vi "GPS Read Sim. Instance.vi"(0 "String In":string, 1 "Buffer In":string, 5 "error in (no error)":errorcluster) -> (13 "Output Valid":bool, 14 "String Out":string, 15 "Buffer Out":string, 16 "Time":dbl, 17 "Longitude":dbl, 18 "Latitude":dbl, 19 "error out":errorcluster)   [LabVIEW 2009]
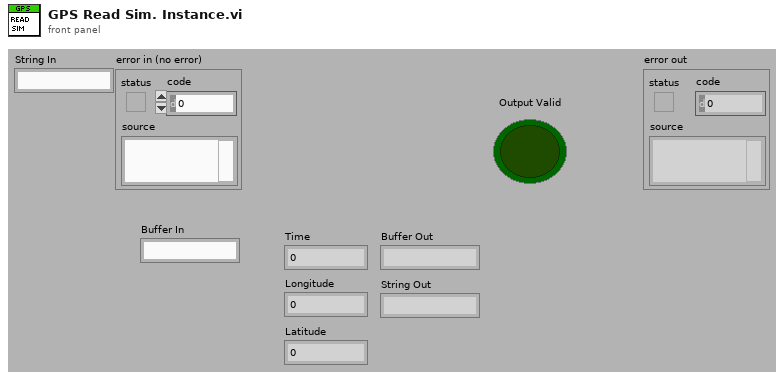
[diagram p1: front panel]
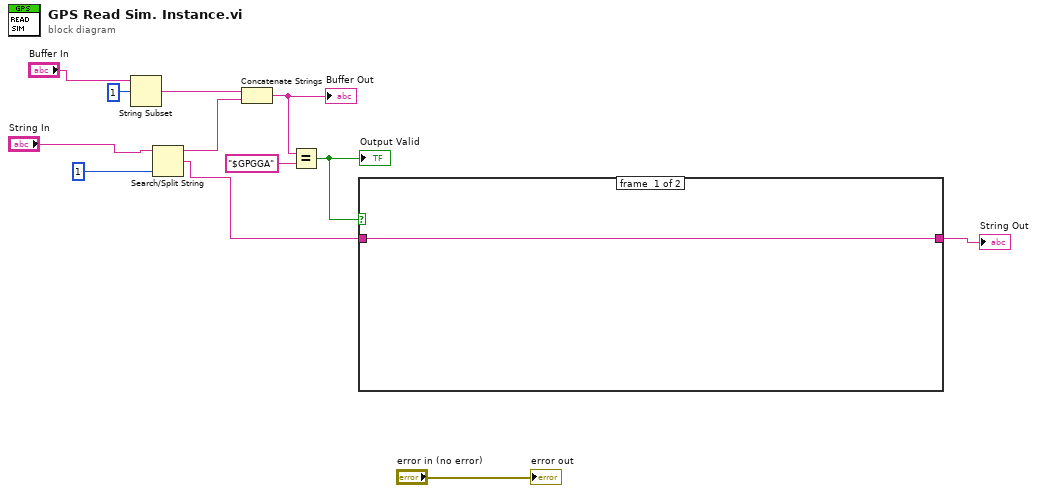
[diagram p0: block diagram]
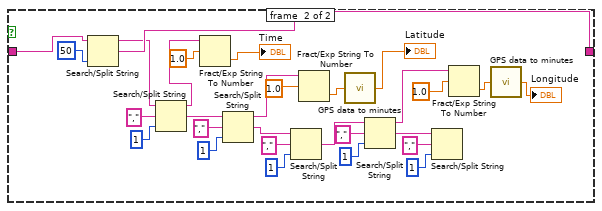
[diagram p2: hidden frame]
diagram:
  n1 = String Subset(string="Buffer In", offset (0)=1) -> (substring=w11:string)  [unwired: 1 in]
  n2 = Search/Split String(string="String In", offset (0)=1 ("length (rest)")) -> (substring before match=w4:string, match + rest of string=w3:string)  [unwired: 1 in, 1 out]
  n3 = Concatenate Strings(w11, w4) -> (w10:string)
  "Buffer Out" <- w10
  n4 = Equal?(x=w10, y="$GPGGA") -> (x = y?=w8:bool)
  "Output Valid" <- w8
  n5 = case shown="True" w8 {
    tunnel: w3 -> [w13 w42]
    tunnel: [w13 w19] -> w2
    frame #0 {
    }
    frame #1 {
      n6 = Search/Split String(string=w42, offset (0)=u32 50 ("byte count")) -> (substring before match=w18:string, match + rest of string=w19:string)  [unwired: 1 in, 1 out]
      n7 = Search/Split String(string=w18, search string/char (-)=",", offset (0)=1) -> (substring before match=w24:string, match + rest of string=w35:string)  [unwired: 1 out]
      n8 = Fract/Exp String To Number(string=w24, offset=1.0 ("default (0 I32)")) -> (number=→"Time":dbl)  [unwired: 2 in, 1 out]
      n9 = Search/Split String(string=w35, search string/char (-)=",", offset (0)=1) -> (substring before match=w27:string, match + rest of string=w34:string)  [unwired: 1 out]
      n10 = Search/Split String(string=w34, search string/char (-)=",", offset (0)=1) -> (match + rest of string=w31:string)  [unwired: 2 out]
      n11 = Fract/Exp String To Number(string=w27, offset=1.0 ("default (0 DBL)")) -> (number=w15:dbl)  [unwired: 2 in, 1 out]
      n12 = call "GPS data to minutes.vi"("GPS Data in (DDmm.mm)"=w15) -> ("GPS Data out (in minutes)"=→"Latitude":dbl)
      n13 = Search/Split String(string=w31, search string/char (-)=",", offset (0)=1) -> (substring before match=w25:string, match + rest of string=w28:string)  [unwired: 1 out]
      n14 = Search/Split String(string=w28, search string/char (-)=",", offset (0)=1) -> ()  [unwired: 3 out]
      n15 = Fract/Exp String To Number(string=w25, offset=1.0 ("default (0 I32)")) -> (number=w16:dbl)  [unwired: 2 in, 1 out]
      n16 = call "GPS data to minutes.vi"("GPS Data in (DDmm.mm)"=w16) -> ("GPS Data out (in minutes)"=→"Longitude":dbl)
    }
  }
  "String Out" <- w2
  "error out" <- "error in (no error)"
